vi "PosesAreClose.vi"(7 "Tolerance":dbl=1.0, 8 "Position 2":T1={"e0"=8.898926, "e1"=45.791016, "s0"=-1.252441, "s1"=-34.541016, "w0"=-12.875977, "w1"=74.750976, "w2"=9.008789} {"w2" scale=-175.25..175.25; "w1" scale=-90.0..120.0; "w0" scale=-175.25..175.25; "e1" scale=-3.0..150.0; "e0" scale=-173.5..173.5; "s1" scale=-123.0..60.0; "s0" scale=-141.0..51.0}, 11 "Position":T1={"e0"=8.898926, "e1"=45.791016, "s0"=-1.252441, "s1"=-34.541016, "w0"=-12.875977, "w1"=74.750976, "w2"=9.008789} {"w2" scale=-175.25..175.25; "w1" scale=-90.0..120.0; "w0" scale=-175.25..175.25; "e1" scale=-3.0..150.0; "e0" scale=-173.5..173.5; "s1" scale=-123.0..60.0; "s0" scale=-141.0..51.0}) -> (1 "Close":bool)   [LabVIEW 2013]
uses:
  ROS/Code/JointPositions.ctl
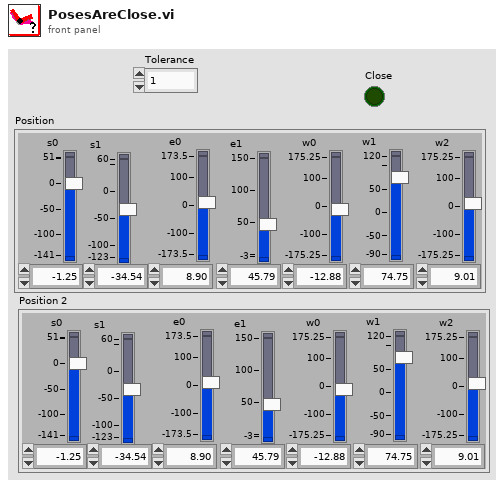
[diagram p1: front panel]
types:
  T1 = typedef "JointPositions.ctl" = cluster{"e0":dbl, "e1":dbl, "s0":dbl, "s1":dbl, "w0":dbl, "w1":dbl, "w2":dbl}
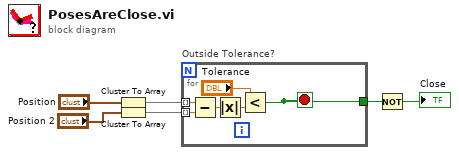
[diagram p0: block diagram]
diagram:
  n1 = Cluster To Array(cluster="Position") -> (array=w5:dbl[])
  n2 = Cluster To Array(cluster="Position 2") -> (array=w4:dbl[])
  n3 = for "Outside Tolerance?" {
    tunnel: w5 -> [w11] mode=indexing
    tunnel: w4 -> [w10] mode=indexing
    tunnel: [w8] -> w2
    stop <- w8 stop-if-true
    n4 = Subtract(x=w11, y=w10) -> (x-y=w12:dbl)
    n5 = Absolute Value(x=w12) -> (abs(x)=w9:dbl)
    n6 = Less?(x="Tolerance", y=w9) -> (x < y?=w8:bool)
  }
  n7 = Not(x=w2) -> (.not. x?=→"Close":bool)
